vi "Get Path Type.vi"(0 "Path in":refnum<class "Path.lvclass">, 11 "error in":errorcluster) -> (4 "Path out":refnum<class "Path.lvclass">, 6 "Path Type":T1, 15 "error out":errorcluster)   [LabVIEW 2023]
uses:
  Common/Base Classes/Path/Path.lvclass
  Type Definitions/Path Types.ctl
  Fixture/Public/Base Classes/Vector/Vector Abstract Path/Vector Abstract Path.lvclass
  C:/rfcal/AuxTools/STSRFFixtureCharactUtility/Source/Code Modules/Common/Base Classes/Path/Path.lvclass
  Fixture/Public/Base Classes/Scalar/SA Abstract Path/SA Abstract Path.lvclass
  Fixture/Public/Base Classes/Scalar/SG Abstract Path/SG Abstract Path.lvclass
  <vilib>/Utility/error.llb/Error Cluster From Error Code.vi
  <vilib>/ErrorRing/Error Ring.xnode
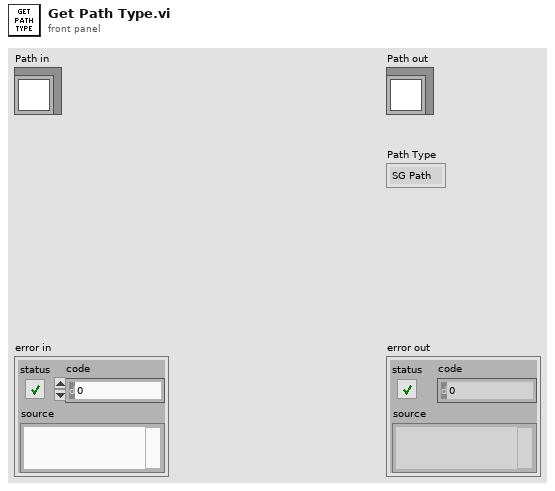
[diagram p1: front panel]
types:
  T1 = typedef "Path Types.ctl" = enum16{"SG Path", "SA Path", "Vector Path"}
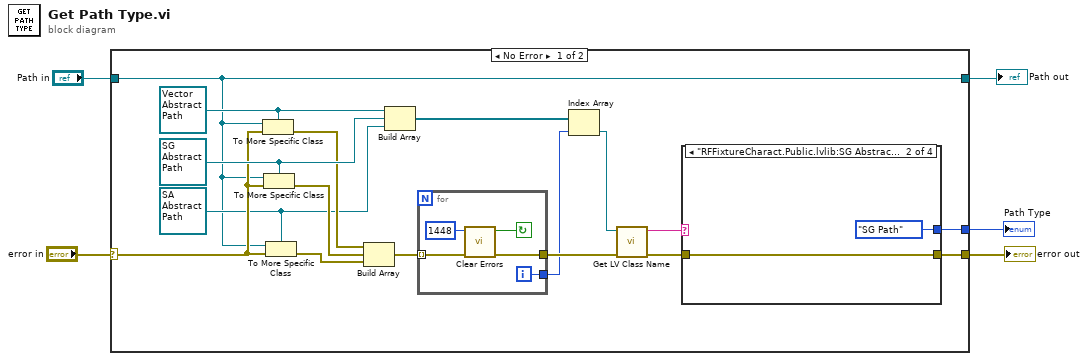
[diagram p0: block diagram]
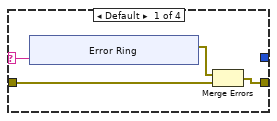
[diagram p2: hidden frame]
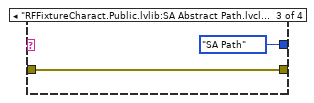
[diagram p3: hidden frame]
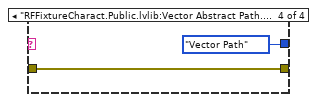
[diagram p4: hidden frame]
diagram:
  n1 = case shown="No Error" "error in" {
    selector: "error in" -> [w12 w46]
    tunnel: "Path in" -> [w6 w45]
    tunnel: [w10 w46] -> w4
    tunnel: [w7 _] -> w2
    tunnel: [w6 w45] -> w1
    frame No Error {
      w21 = refnum<class "SG Abstract Path.lvclass"> refnum ("RFFixtureCharact.Public.lvlib:SG Abstract Path.lvclass")
      w8 = refnum<class "SA Abstract Path.lvclass"> refnum ("RFFixtureCharact.Public.lvlib:SA Abstract Path.lvclass")
      w22 = refnum<class "Vector Abstract Path.lvclass"> refnum ("RFFixtureCharact.Public.lvlib:Vector Path.lvclass")
      n2 = To More Specific Class(target class=w22, reference=w6, error in=w12) -> (error out=w13:errorcluster)  [unwired: 1 out]
      n3 = To More Specific Class(target class=w21, reference=w6, error in=w12) -> (error out=w14:errorcluster)  [unwired: 1 out]
      n4 = To More Specific Class(target class=w8, reference=w6, error in=w12) -> (error out=w15:errorcluster)  [unwired: 1 out]
      n5 = Build Array(w13, w14, w15) -> (w16:errorcluster[])
      n6 = Build Array(w22, w21, w8) -> (w17:refnum<class "Path.lvclass">[])
      n7 = for {
        tunnel: w16 -> [w27] mode=indexing
        tunnel: [w25] -> w19
        tunnel: [w24] -> w18
        i -> [w24]
        stop <- w26 continue-if-true
        n8 = call <vilib>:"Clear Errors.vi"("error in (no error)"=w27, "specific error code to clear (0: all)"=1448) -> ("error out"=w25:errorcluster, "specific error cleared?"=w26:bool)  [unwired: 4 in]
      }
      n9 = Index Array(array=w17, index=w18) -> (element=w20:refnum<class "Path.lvclass">)
      n10 = call <vilib>:"Get LV Class Name.vi"("error in (no error)"=w19, "object"=w20) -> ("error out"=w9:errorcluster, "class name"=w11:string)  [unwired: 8 in]
      n11 = case shown="\"RFFixtureCharact.Public.lvlib:SG Abstract Path.lvclass\"" w11 {
        selector: w11 -> [w28 _ _ _]
        tunnel: [w31 w40 w42 w44] -> w10
        tunnel: w9 -> [w30 w40 w42 w44]
        tunnel: [_ Path_Types."SG Path" ("Path Type") Path_Types."SA Path" ("Path Type") Path_Types."Vector Path" ("Path Type")] -> w7
        frame Default {
          n12 = xnode "Error Ring"("parameter 0"=w28) -> ("error out"=w29:errorcluster)
          n13 = Merge Errors(w29, w30) -> (w31:errorcluster)
        }
        frame "RFFixtureCharact.Public.lvlib:SG Abstract Path.lvclass" {
        }
        frame "RFFixtureCharact.Public.lvlib:SA Abstract Path.lvclass" {
        }
        frame "RFFixtureCharact.Public.lvlib:Vector Abstract Path.lvclass" {
        }
      }
    }
    frame Error {
    }
  }
  "error out" <- w4
  "Path Type" <- w2
  "Path out" <- w1
